vi "From Serial Form.vi"(6 "Serial Version":T1, 10 "Deserializer in":refnum<class "Deserializer.lvclass">=refnum, 11 "Switch in":refnum<class "Switch.lvclass">) -> (0 "error out":errorcluster, 2 "Deserializer out":refnum<class "Deserializer.lvclass">, 3 "Switch out":refnum<class "Switch.lvclass">)   [LabVIEW 2014]
uses:
  <userlib>/Serialization/Serializable/Remove Double.vi
  <userlib>/Serialization/Serializable/Remove Boolean.vi
  <userlib>/Serialization/Serialization Common/Serial Version.ctl
  <userlib>/Serialization/Deserializer/Deserializer.lvclass
  Switch.lvclass
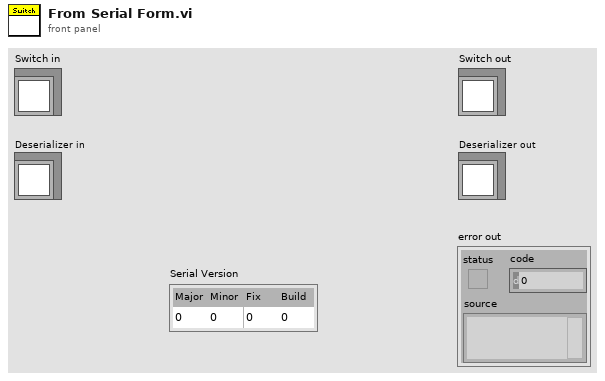
[diagram p1: front panel]
types:
  T1 = typedef "Serialization Common.lvlib/Serial Version.ctl" = cluster{"Major":u16, "Minor":u16, "Fix":u16, "Build":u16}
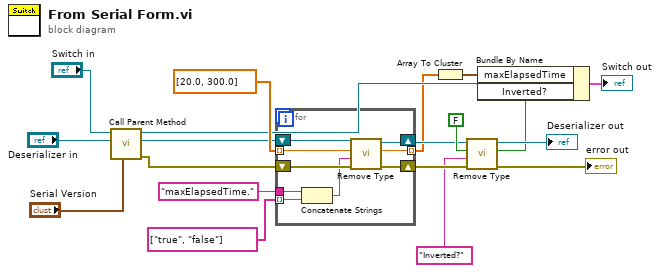
[diagram p0: block diagram]
diagram:
  n1 = call-parent "Call Parent Method"("Serial Version"="Serial Version", "Deserializer in"="Deserializer in", "Serializable in"="Switch in") -> ("error out"=w1:errorcluster, "Deserializer out"=w13:refnum<class "Deserializer.lvclass">, "Serializable out"=w7:refnum<class "Serializable.lvclass">)  [unwired: 6 in]
  n2 = for {
    tunnel: string[] ["true", "false"] -> [w28] mode=indexing
    tunnel: "maxElapsedTime." ("string") -> [w27]
    tunnel: dbl[] [20.0, 300.0] -> [w21] mode=indexing
    shift-right: [w24] -> w10
    shift-left: w1 -> [w23]
    tunnel: [w20] -> w5 mode=indexing
    shift-right: [w25] -> w11
    shift-left: w13 -> [w26]
    n3 = Concatenate Strings(w27, w28) -> (w22:string)
    n4 = call-poly <userlib>:"Remove Type.vi"("error in (no error)"=w23, "Name"=w22, "Default Value"=w21, "Deserializer in"=w26) -> ("error out"=w24:errorcluster, "Numeric"=w20:dbl, "Deserializer out"=w25:refnum<class "Deserializer.lvclass">)  [unwired: 4 in, 1 out]
  }
  n5 = Array To Cluster(array=w5) -> (cluster=w4:cluster{"[0]":dbl, "[1]":dbl})
  n6 = call-poly <userlib>:"Remove Type.vi"("error in (no error)"=w10, "Name"="Inverted?", "Default Value"=FALSE, "Deserializer in"=w11) -> ("error out"=→"error out":errorcluster, "Boolean"=w6:bool, "Deserializer out"=→"Deserializer out":refnum<class "Deserializer.lvclass">)  [unwired: 4 in, 1 out]
  n7 = Bundle By Name(cluster=w7, "maxElapsedTime"=w4, "Inverted?"=w6) -> (→"Switch out":cluster{})
